vi "Read Comment.vi"(8 "error in (no error)":errorcluster, 11 "Save Image in":refnum<class "Save Image.lvclass">) -> (0 "error out":errorcluster, 2 "COMMENT.Value":string, 3 "Save Image out":refnum<class "Save Image.lvclass">)   [LabVIEW 2018, in "Save Image.lvclass"]
uses:
  Save Image.lvclass
  Simulated_Header/Simulated_Header.lvclass
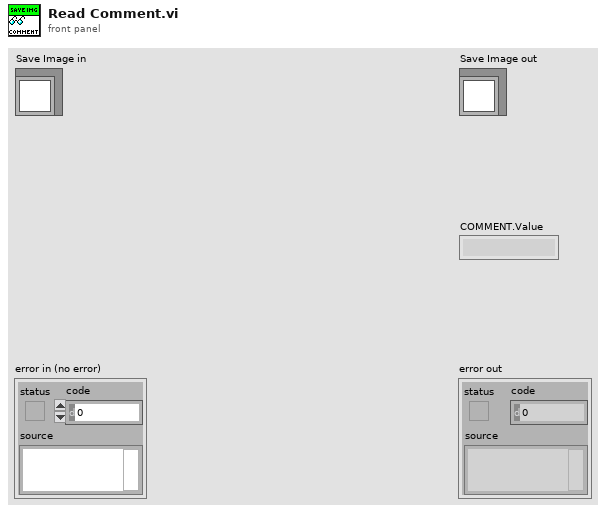
[diagram p1: front panel]
types:
  T1 = cluster{"FILENAME":cluster{"Name":string, "Value":string, "Comment":string}, "OBSERVER":cluster{"Name":string, "Value":string, "Comment":string}, "PROGRID":cluster{"Name":string, "Value":string, "Comment":string}, "OBJECT":cluster{"Name":string, "Value":string, "Comment":string}, "NIGHTDIR":cluster{"Name":string, "Value":string, "Comment":string}, "CHANNEL":cluster{"Name":string, "Value":string, "Comment":string}, "INSTRUME":cluster{"Name":string, "Value":string, "Comment":string}, "NEXPSEQ":cluster{"Name":string, "Value":u16, "Comment":string}, "SEQINDEX":cluster{"Name":string, "Value":u16, "Comment":string}, "OBSTYPE":cluster{"Name":string, "Value":string, "Comment":string}, "READMOD":cluster{"Name":string, "Value":string, "Comment":string}, "READMODE":cluster{"Name":string, "Value":string, "Comment":string}, "ACQMODE":cluster{"Name":string, "Value":string, "Comment":string}, "PREAMP":cluster{"Name":string, "Value":string, "Comment":string}, "READOUT":cluster{"Name":string, "Value":string, "Comment":string}, "VSHIFT":cluster{"Name":string, "Value":string, "Comment":string}, "TRIGGER":cluster{"Name":string, "Value":string, "Comment":string}, "EMMODE":cluster{"Name":string, "Value":string, "Comment":string}, "EMGAIN":cluster{"Name":string, "Value":u16, "Comment":string}, "VBIN":cluster{"Name":string, "Value":u16, "Comment":string}, "HBIN":cluster{"Name":string, "Value":u16, "Comment":string}, "INITLIN":cluster{"Name":string, "Value":u16, "Comment":string}, "INITCOL":cluster{"Name":string, "Value":u16, "Comment":string}, "FINALLIN":cluster{"Name":string, "Value":u16, "Comment":string}, "FINALCOL":cluster{"Name":string, "Value":u16, "Comment":string}, "KSERLEN":cluster{"Name":string, "Value":u16, "Comment":string}, "SHUTTER":cluster{"Name":string, "Value":string, "Comment":string}, "OPENSHT":cluster{"Name":string, "Value":u16, "Comment":string}, "CLOSESHT":cluster{"Name":string, "Value":u16, "Comment":string}, "DATE":cluster{"Name":string, "Value":string, "Comment":string}, "GAIN":cluster{"Name":string, "Value":dbl, "Comment":string}, "GAINERR":cluster{"Name":string, "Value":dbl, "Comment":string}, "RDNOISE":cluster{"Name":string, "Value":dbl, "Comment":string}, "RNOISERR":cluster{"Name":string, "Value":dbl, "Comment":string}, "SKYFIBER":cluster{"Name":string, "Value":string, "Comment":string}, "CALFIBER":cluster{"Name":string, "Value":string, "Comment":string}, "UTDATE":cluster{"Name":string, "Value":string, "Comment":string}, "LOCTIME":cluster{"Name":string, "Value":string, "Comment":string}, "MJD":cluster{"Name":string, "Value":dbl, "Comment":string}, "OBSLON":cluster{"Name":string, "Value":string, "Comment":string}, "OBSLAT":cluster{"Name":string, "Value":string, "Comment":string}, "OBSALT":cluster{"Name":string, "Value":dbl, "Comment":string}, "EXPTIME":cluster{"Name":string, "Value":dbl, "Comment":string}, "TELRA":cluster{"Name":string, "Value":string, "Comment":string}, "TELDEC":cluster{"Name":string, "Value":string, "Comment":string}, "RA":cluster{"Name":string, "Value":string, "Comment":string}, "DEC":cluster{"Name":string, "Value":string, "Comment":string}, "RA_DEG":cluster{"Name":string, "Value":dbl, "Comment":string}, "DEC_DEG":cluster{"Name":string, "Value":dbl, "Comment":string}, "EPOCH":cluster{"Name":string, "Value":dbl, "Comment":string}, "HA":cluster{"Name":string, "Value":string, "Comment":string}, "HAD":cluster{"Name":string, "Value":dbl, "Comment":string}, "AIRMASS":cluster{"Name":string, "Value":dbl, "Comment":string}, "AMSTART":cluster{"Name":string, "Value":dbl, "Comment":string}, "AMEND":cluster{"Name":string, "Value":dbl, "Comment":string}, "XOFFSET":cluster{"Name":string, "Value":dbl, "Comment":string}, "YOFFSET":cluster{"Name":string, "Value":dbl, "Comment":string}, "PA":cluster{"Name":string, "Value":dbl, "Comment":string}, "CAMFOC":cluster{"Name":string, "Value":string, "Comment":string}, "TELFOC":cluster{"Name":string, "Value":dbl, "Comment":string}, "TCSUT":cluster{"Name":string, "Value":string, "Comment":string}, "TCSST":cluster{"Name":string, "Value":string, "Comment":string}, "MOONDIST":cluster{"Name":string, "Value":dbl, "Comment":string}, "MOONALT":cluster{"Name":string, "Value":dbl, "Comment":string}, "MOONPHAS":cluster{"Name":string, "Value":string, "Comment":string}, "ADC":cluster{"Name":string, "Value":string, "Comment":string}, "ADCSPEED":cluster{"Name":string, "Value":dbl, "Comment":string}, "CALMIRR":cluster{"Name":string, "Value":string, "Comment":string}, "GUIDING":cluster{"Name":string, "Value":string, "Comment":string}, "GUIDTEXP":cluster{"Name":string, "Value":dbl, "Comment":string}, "GUIDFREQ":cluster{"Name":string, "Value":dbl, "Comment":string}, "GUIDOBJX":cluster{"Name":string, "Value":dbl, "Comment":string}, "GUIDOBJY":cluster{"Name":string, "Value":dbl, "Comment":string}, "AVGYCORR":cluster{"Name":string, "Value":dbl, "Comment":string}, "AVGXCORR":cluster{"Name":string, "Value":dbl, "Comment":string}, "GFOCUS":cluster{"Name":string, "Value":dbl, "Comment":string}, "THARLAMP":cluster{"Name":string, "Value":string, "Comment":string}, "HALLAMP":cluster{"Name":string, "Value":string, "Comment":string}, "AGITATOR":cluster{"Name":string, "Value":string, "Comment":string}, "THARMIRR":cluster{"Name":string, "Value":string, "Comment":string}, "DSTATUS":cluster{"Name":string, "Value":string, "Comment":string}, "DPOS":cluster{"Name":string, "Value":dbl, "Comment":string}, "DTEMP":cluster{"Name":string, "Value":dbl, "Comment":string}, "DHUM":cluster{"Name":string, "Value":string, "Comment":string}, "DLAMP":cluster{"Name":string, "Value":string, "Comment":string}, "DFLAT":cluster{"Name":string, "Value":string, "Comment":string}, "TEMPEXT":cluster{"Name":string, "Value":string, "Comment":string}, "PRESSURE":cluster{"Name":string, "Value":string, "Comment":string}, "HUMIDITY":cluster{"Name":string, "Value":string, "Comment":string}, "WINDDIR":cluster{"Name":string, "Value":string, "Comment":string}, "WINSPEED":cluster{"Name":string, "Value":dbl, "Comment":string}, "SHTTTL":cluster{"Name":string, "Value":string, "Comment":string}, "COOLER":cluster{"Name":string, "Value":string, "Comment":string}, "TEMP":cluster{"Name":string, "Value":u16, "Comment":string}, "TEMPST":cluster{"Name":string, "Value":string, "Comment":string}, "SERN":cluster{"Name":string, "Value":u16, "Comment":string}, "COMMENT":cluster{"Name":string, "Value":string, "Comment":string}, "SIMPLE":cluster{"Name":string, "Value":string, "Comment":string}, "BITPIX":cluster{"Name":string, "Value":u16, "Comment":string}, "NAXIS":cluster{"Name":string, "Value":u16, "Comment":string}, "EXTEND":cluster{"Name":string, "Value":string, "Comment":string}, "FRAME_T":cluster{"Name":string, "Value":string, "Comment":string}, "VCLOCK":cluster{"Name":string, "Value":string, "Comment":string}, "ADCHNNL":cluster{"Name":string, "Value":u16, "Comment":string}, "JD":cluster{"Name":string, "Value":dbl, "Comment":string}, "SD":cluster{"Name":string, "Value":string, "Comment":string}, "FILTER":cluster{"Name":string, "Value":string, "Comment":string}}
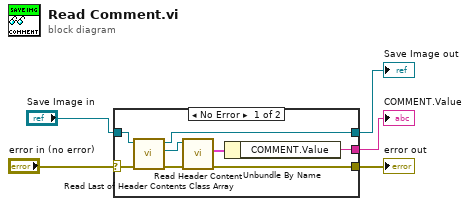
[diagram p0: block diagram]
diagram:
  n1 = case shown="No Error" "error in (no error)" {
    selector: "error in (no error)" -> [w11 w15]
    tunnel: [w7 w15] -> w4
    tunnel: [w10 w14] -> w2
    tunnel: "Save Image in" -> [w12 w14]
    tunnel: [w13 _] -> w1
    frame No Error {
      n2 = call "Read Last of Header Contents Class Array.vi"("error in (no error)"=w11, "Save Image in"=w12) -> ("error out"=w6:errorcluster, "Simulated_Header.lvclass"=w9:refnum<class "Simulated_Header.lvclass">, "Save Image out"=w10:refnum<class "Save Image.lvclass">)  [unwired: 7 in]
      n3 = call "Read Header Content.vi"("error in (no error)"=w6, "Simulated_Header in"=w9) -> ("error out"=w7:errorcluster, "Header Content"=w8:T1)  [unwired: 7 in, 1 out]
      n4 = Unbundle By Name(w8) -> ("COMMENT.Value"=w13:string)
    }
    frame Error {
    }
  }
  "error out" <- w4
  "Save Image out" <- w2
  "COMMENT.Value" <- w1
